vi "To JSON - Warning Input - Returns Same Warning.vi"() -> ()   [LabVIEW 2017, in "JSON Serializable Tests.lvlib"]
uses:
  JSON Serializable Tests.lvlib
  JSON Serializable/JSON Serializable.lvclass
  <vilib>/JDP Science/JSONtext/LVClass Serializer/JSONtext LVClass Serializer.lvclass
  <vilib>/Utility/error.llb/Error Cluster From Error Code.vi
  <vilib>/addons/_JKI Toolkits/Caraya/classes/Assert/Assert Equal Value_Variant.vi
  <vilib>/ErrorRing/Error Ring.xnode
  <vilib>/addons/_JKI Toolkits/Caraya/classes/Test/Test.lvclass
  <vilib>/addons/_JKI Toolkits/Caraya/classes/Assert/Assert.lvclass
panel:
  out "error out":errorcluster
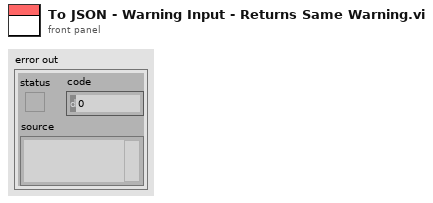
[diagram p1: front panel]
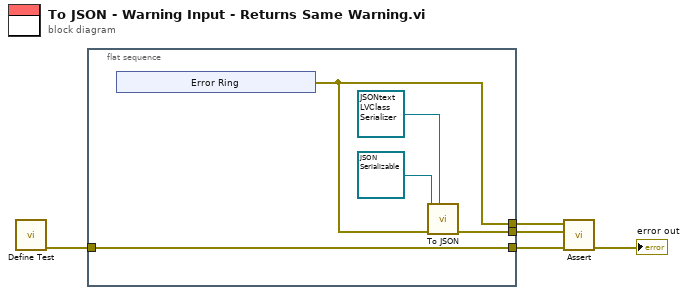
[diagram p0: block diagram]
diagram:
  n1 = call <vilib>:"Define Test.vi"() -> ("error out"=w2:errorcluster)  [unwired: 11 in]
  n2 = flat-sequence {
    tunnel: [w9] -> w5
    tunnel: [w8] -> w4
    tunnel: [w7] -> w3
    tunnel: w2 -> [w7]
    frame #0 {
      n3 = xnode "Error Ring"() -> ("error out"=w8:errorcluster)
      n4 = call-dynamic "To JSON.vi"("LVClass Serializer"=refnum<class "JSONtext LVClass Serializer.lvclass"> refnum, "error in (no error)"=w8, "JSON Serializable in"=refnum<class "JSON Serializable.lvclass"> refnum ("JSON Serializable.lvclass")) -> ("error out"=w9:errorcluster)  [unwired: 6 in, 2 out]
    }
  }
  n5 = call-poly <vilib>:"Assert.vi"("error in (no error)"=w3, "Y"=w5, "X"=w4) -> ("error out"=→"error out":errorcluster)  [unwired: 8 in]
